vi "CLSUIP_GetProjItemOfMemberVI.vi"(3 "error in (no error)":errorcluster, 4 "Member Name":string, 5 "Class in":refnum<vi>) -> (0 "error out":errorcluster, 1 "ProjectItem":refnum<vi>, 2 "Class out":refnum<vi>)   [LabVIEW 2021, in "MemberVICreation.lvlib" / "VIRetooler.lvclass"]
uses:
  <resource>/Framework/Providers/LVClassLibrary/NewAccessors/VIRetooler/VIRetooler.lvclass
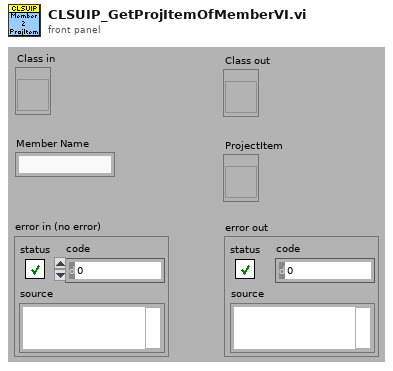
[diagram p1: front panel]
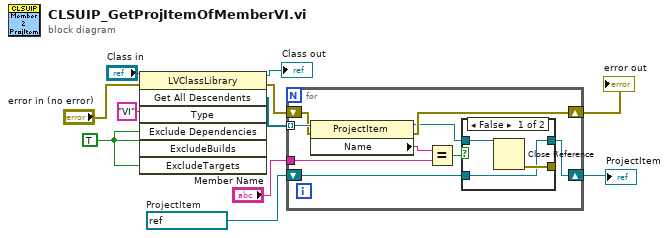
[diagram p0: block diagram]
diagram:
  w2 = refnum<vi> refnum  # ProjectItem
  w6 = TRUE ("ExcludeDependencies")
  n1 = invoke class="LVClassLibrary" method="Get All Descendents"(reference="Class in", error in="error in (no error)", "Type"="VI", "Exclude Dependencies"=w6, "ExcludeBuilds"=w6, "ExcludeTargets"=w6) -> (reference out=→"Class out":refnum<vi>, error out=w8:errorcluster, "All Descendents"=w7:refnum<vi>[])  [unwired: 1 in, 4 out]
  n2 = for {
    tunnel: w7 -> [w20] mode=indexing
    shift-right: [w16] -> w11
    shift-left: w8 -> [w19]
    tunnel: "Member Name" -> [w17]
    shift-right: [w13] -> w10
    shift-left: w2 -> [w12]
    n3 = property class="ProjectItem"(reference=w20, error in=w19) -> (reference out=w14:refnum<vi>, error out=w16:errorcluster, "Name"=w18:string)
    n4 = Equal?(x=w18, y=w17) -> (x = y?=w15:bool)
    n5 = case shown="False" w15 {
      tunnel: w14 -> [w23 w24]
      tunnel: [w21 w24] -> w13
      tunnel: [w22 _] -> _
      tunnel: w12 -> [w21 _]
      frame False {
        n6 = Close Reference(reference=w23) -> (error out=w22:errorcluster)  [unwired: 1 in]
      }
      frame True {
      }
    }
  }
  "error out" <- w11
  "ProjectItem" <- w10
